vi "Get PGI Attribute.vi"(7 "value":u32, 8 "error in (no error)":errorcluster caption="错误输入（无错误）", 9 "attribute":i32, 10 "pgiPort":i32, 11 "pgiType":i32) -> (0 "error out":errorcluster caption="错误输出", 3 "function return":i32, 5 "value out":u32)   [LabVIEW 2018]
doc: "extern int APSxSetPGIAttribute (int pgiType, int pgiDevNum, IN int attribute, IN ...); extern int __stdcall APSxGetPGIAttribute (int pgiType, int pgiPort, IN int attribute, OUT void * value);"
uses:
  APSx.dll/APSx.dll
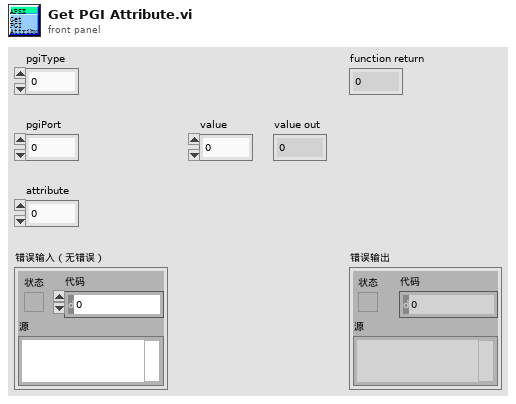
[diagram p1: front panel]
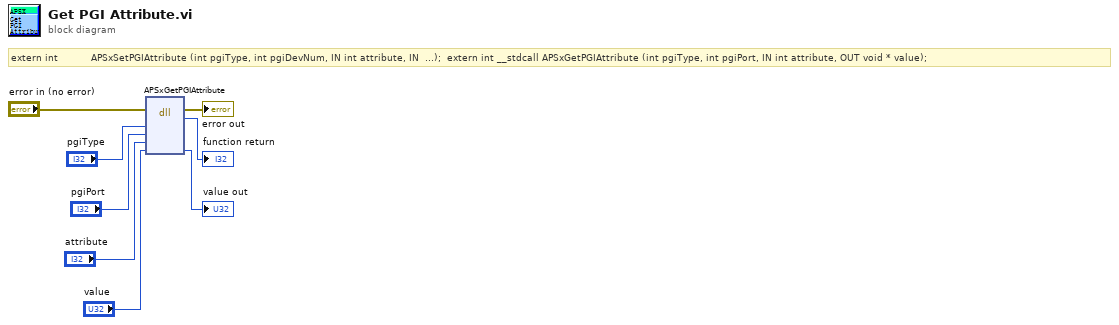
[diagram p0: block diagram]
diagram:
  # "extern int           APSxSetPGIAttribute (int pgiType, int pgiDevNum, IN int attribute, IN  ...);  extern int __stdcall APSxGetPGIAttribute (int pgiType, int pgiPort, IN int attribute, OUT void * value);"
  n1 = dll-call lib="PTH2[abs D项目Feng恒隆项目Labview传感器对中台SourcesAPSx.dllAPSx.*" fn="APSxGetPGIAttribute"(error in="error in (no error)", "pgiType"="pgiType", "pgiPort"="pgiPort", "attribute"="attribute", "value"="value") -> (error out=→"error out":errorcluster, →"function return":i32, "value"=→"value out":u32)  [unwired: 5 in, 1 out]
